vi "test - Apply Exclusion Value - 3.vi"(8 "error in (no error)":errorcluster, 11 "TestCase in":refnum<class "Base Filter Tester.lvclass">) -> (0 "error out":errorcluster, 3 "TestCase out":refnum<class "Base Filter Tester.lvclass">)   [LabVIEW 2016, in "Base Filter Tester.lvclass"]
uses:
  Base Filter Tester.lvclass
  <vilib>/addons/_JKI Toolkits/VI Tester/TestCase.llb/TestCase.lvclass
  Core/Assert API Components/Filter Configurations/Base Filter.lvclass
  C:/Program Files (x86)/National Instruments/LabVIEW 2016/vi.lib/addons/_JKI Toolkits/VI Tester/TestCase.llb/TestCase.lvclass
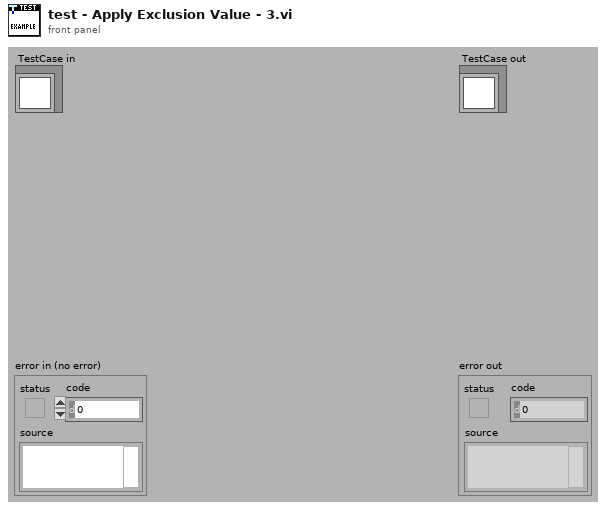
[diagram p1: front panel]
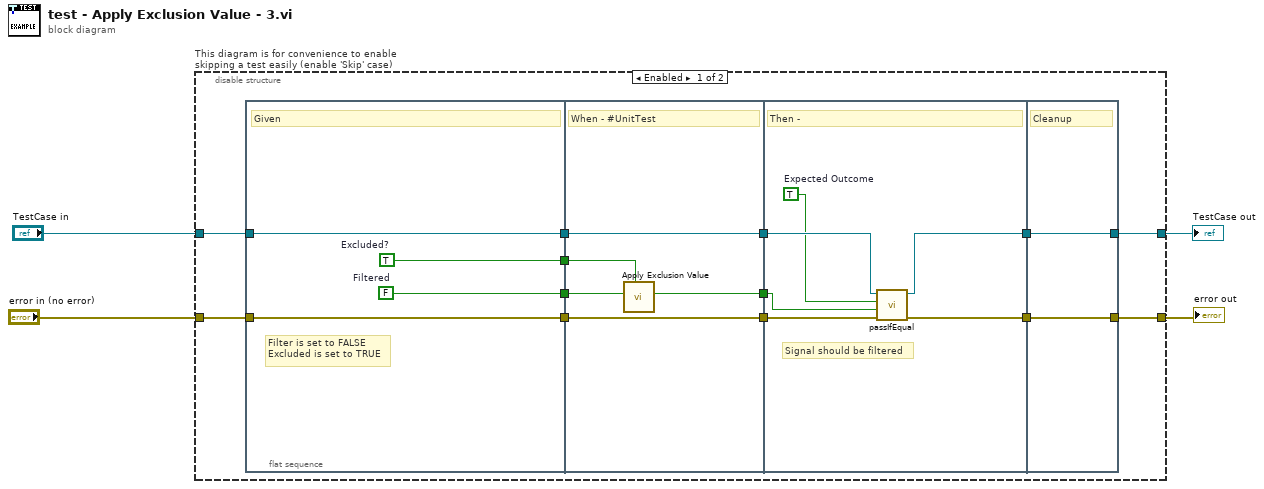
[diagram p0: block diagram]
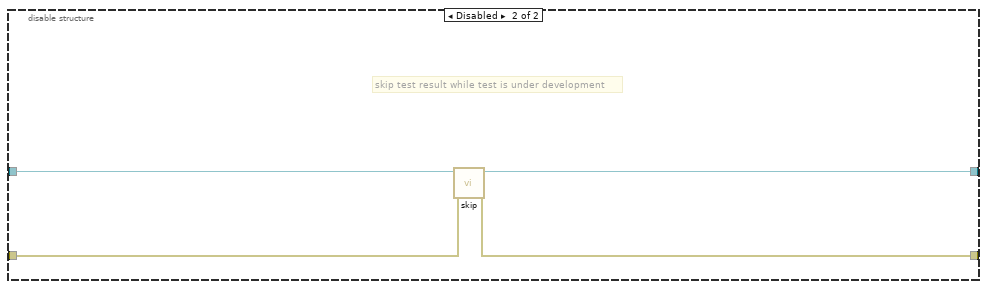
[diagram p2: hidden frame]
diagram:
  n1 = disable-structure "This diagram is for convenience to enable skipping a test easily (enable 'Skip' case)" shown="Enabled" {
    disable-tunnel: "TestCase in" -> [w11 w38]
    disable-tunnel: [w8 w36] -> w1
    disable-tunnel: [w9 w37] -> w3
    disable-tunnel: "error in (no error)" -> [w10 w35]
    frame Enabled {
      n2 = flat-sequence {
        tunnel: w10 -> [w20]
        tunnel: w11 -> [w21]
        tunnel: [w21] -> w17
        tunnel: [w20] -> w16
        tunnel: [w19] -> w7
        tunnel: [w18] -> w6
        tunnel: [w26] -> w15
        tunnel: [w25] -> w14
        tunnel: w17 -> [w26]
        tunnel: w16 -> [w25]
        tunnel: w7 -> [w24]
        tunnel: w6 -> [w23]
        tunnel: [w22] -> w5
        tunnel: [w31] -> w13
        tunnel: [w29] -> w12
        tunnel: w15 -> [w32]
        tunnel: w14 -> [w30]
        tunnel: w5 -> [w28]
        tunnel: [w33] -> w9
        tunnel: [w34] -> w8
        tunnel: w13 -> [w34]
        tunnel: w12 -> [w33]
        frame #0 {
          w19 = FALSE  # Filtered
          w18 = TRUE  # Excluded?
          # "Filter is set to FALSE\nExcluded is set to TRUE"
          # "Given"
        }
        frame #1 {
          # "When - #UnitTest"
          n3 = call "Apply Exclusion Value.vi"("Excluded?"=w23, "Filtered value in"=w24) -> ("Final Filtered Value"=w22:bool)  [unwired: 9 in]
        }
        frame #2 {
          w27 = TRUE  # Expected Outcome
          # "Signal should be filtered"
          # "Then -"
          n4 = call-dynamic "passIfEqual.vi"("error in (no error)"=w30, "y"=w28, "x"=w27, "TestCase in"=w32) -> ("error out"=w29:errorcluster, "TestCase out"=w31:refnum<class "Base Filter Tester.lvclass">)  [unwired: 6 in]
        }
        frame #3 {
          # "Cleanup"
        }
      }
    }
    frame Disabled {
      # "skip test result while test is under development"
      n5 = call <vilib>:"skip.vi"("error in (no error)"=w35, "TestCase in"=w38) -> ("error out"=w37:errorcluster, "TestCase out"=w36:refnum<class "Base Filter Tester.lvclass">)  [unwired: 8 in]
    }
  }
  "error out" <- w3
  "TestCase out" <- w1
